vi "Set Tray Icon Tip Strip.vi"(0 "NotifyIcon in":refnum<class "NotifyIcon.lvclass">, 7 "Icon Tip Strip Text":string, 11 "error in (no error)":errorcluster) -> (4 "NotifyIcon out":refnum<class "NotifyIcon.lvclass">, 15 "error out":errorcluster)   [LabVIEW 2016, in "NotifyIcon.lvclass"]
doc: "This VI sets the text string that is displayed when the user hoovers the mouse on the Tray Icon associated with the Notification Icon.\n\n\nStinus Olsen\nCIM Industrial Systems A/S\n22. Feb. 2011 15:06\nmailto: seo@cim.as"
uses:
  NotifyIcon.lvclass
  NotifyIcon.lvclass/NotifyIcon.ctl
  System.Windows.Forms
panel:
  # "This VI belongs to the NotifyIcon Toolset. \nA toolset that makes it easy to create, control and manipulate a notification icon in the notification area of the Windows taskbar.\nThe toolset requires Microsoft .NET framework 2.0\n\n\nNOTICE -- YOU MUST LEAVE THIS NOTICE IN PLACE.  PER THE TERMS OF THE LICENSE BELOW, YOU MAY SUBLICENSE THIS SOFTWARE \nIN ANY WAY THAT DOES NOT CONFLICT WITH THIS LICENSE.\n\n### BSD License (http://www.opensource.org/licenses/bsd-license.php) Begin ###\n \nCopyright (c) 2011, Stinus Olsen <seo@cim.as>\n\nAll rights reserved.\n\nRedistribution and use in source and binary forms, with or without modification, are permitted provided that the following conditions are met:\n\n    * Redistributions of source code must retain the above copyright notice, this list of conditions and the following disclaimer.\n    * Redistributions in binary form must reproduce the above copyright notice, this list of conditions and the following disclaimer in the \n       documentation and/or other materials provided with the distribution.\n    * Neither the name of CIM Industrial Systems nor the names of its contributors may be used to endorse or promote products derived \n       from this software without specific prior written permission.\n\nTHIS SOFTWARE IS PROVIDED BY THE COPYRIGHT HOLDERS AND CONTRIBUTORS \"AS IS\" AND ANY EXPRESS OR IMPLIED WARRANTIES, \nINCLUDING, BUT NOT LIMITED TO, THE IMPLIED WARRANTIES OF MERCHANTABILITY AND FITNESS FOR A PARTICULAR PURPOSE ARE \nDISCLAIMED. IN NO EVENT SHALL THE COPYRIGHT OWNER OR CONTRIBUTORS BE LIABLE FOR ANY DIRECT, INDIRECT, INCIDENTAL,\n SPECIAL, EXEMPLARY, OR CONSEQUENTIAL DAMAGES (INCLUDING, BUT NOT LIMITED TO, PROCUREMENT OF SUBSTITUTE GOODS OR \nSERVICES; LOSS OF USE, DATA, OR PROFITS; OR BUSINESS INTERRUPTION) HOWEVER CAUSED AND ON ANY THEORY OF LIABILITY, \nWHETHER IN CONTRACT, STRICT LIABILITY, OR TORT (INCLUDING NEGLIGENCE OR OTHERWISE) ARISING IN ANY WAY OUT OF THE USE \nOF THIS SOFTWARE, EVEN IF ADVISED OF THE POSSIBILITY OF SUCH DAMAGE.\n\n### BSD License End ###"
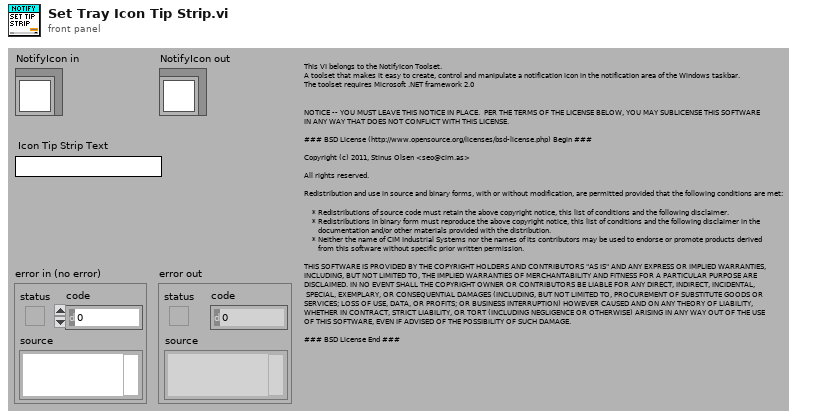
[diagram p1: front panel]
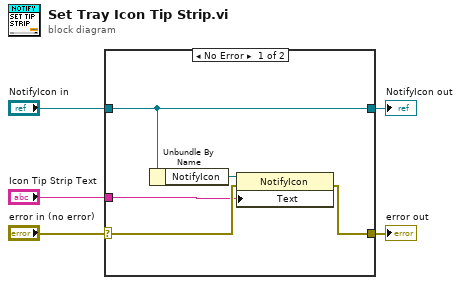
[diagram p0: block diagram]
diagram:
  n1 = case shown="No Error" "error in (no error)" {
    selector: "error in (no error)" -> [w8 w12]
    tunnel: [w7 w12] -> w4
    tunnel: [w10 w11] -> w2
    tunnel: "NotifyIcon in" -> [w10 w11]
    tunnel: "Icon Tip Strip Text" -> [w6 _]
    frame No Error {
      n2 = Unbundle By Name(w10) -> ("NotifyIcon"=w9:refnum<k24>)
      n3 = property class="NotifyIcon"(reference=w9, error in=w8, "Text"=w6) -> (error out=w7:errorcluster)  [unwired: 1 out]
    }
    frame Error {
    }
  }
  "error out" <- w4
  "NotifyIcon out" <- w2
